vi "_Template Read sqlite configuration.vi"(8 "error in (no error)":errorcluster, 10 "Table in":string="employees", 11 "Configuration database in":path) -> (0 "error out":errorcluster, 1 "Values(str)":string[](array[string]), 2 "Names":string[](array[string]))   [LabVIEW 2020, in "sqlite3.lvlib" / "sqlite3.lvclass"]
uses:
  externals/sqlite3/Source/sqlite3.lvclass
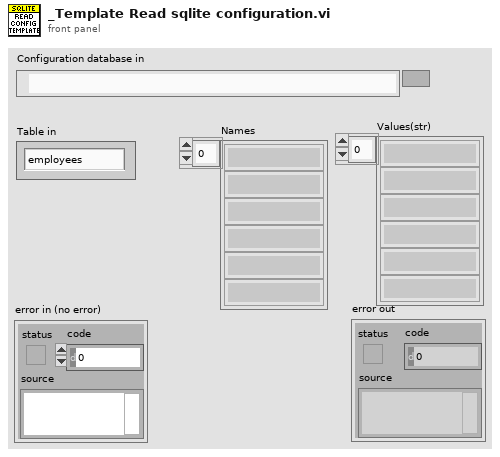
[diagram p1: front panel]
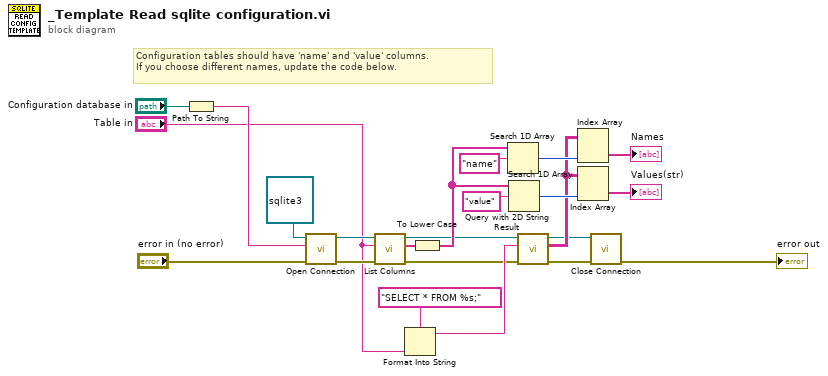
[diagram p0: block diagram]
diagram:
  # "Configuration tables should have 'name' and 'value' columns.\nIf you choose different names, update the code below."
  n1 = Path To String(path="Configuration database in") -> (string=w20:string)
  n2 = call-dynamic "Open Connection.vi"("error in (no error)"="error in (no error)", "DatabaseFilePath"=w20, "sqlite in"=refnum<class "sqlite3.lvclass"> refnum) -> ("error out"=w16:errorcluster, "sqlite out"=w17:refnum<class "sqlite3.lvclass">)  [unwired: 7 in]
  n3 = call-dynamic "List Columns.vi"("error in (no error)"=w16, "Table in"="Table in", "sqlite in"=w17) -> ("error out"=w4:errorcluster, "columns out"=w13:string[], "sqlite out"=w6:refnum<class "sqlite3.lvclass">)  [unwired: 5 in, 1 out]
  n4 = Format Into String(format string="SELECT * FROM %s;" ("sql (string)"), "Table in") -> (resulting string=w5:string)  [unwired: 2 in, 1 out]
  n5 = To Lower Case(string=w13) -> (all lower case string=w11:string[])
  n6 = Search 1D Array(1D array=w11, element="name" ("sql (string)")) -> (index of element=w10:i32)  [unwired: 1 in]
  n7 = Search 1D Array(1D array=w11, element="value" ("sql (string)")) -> (index of element=w9:i32)  [unwired: 1 in]
  n8 = call-dynamic "Query with 2D String Result.vi"("error in (no error)"=w4, "Query string"=w5, "sqlite3 in"=w6) -> ("error out"=w1:errorcluster, "Result"=w3:string[][], "sqlite3 out"=w2:refnum<class "sqlite3.lvclass">)  [unwired: 6 in]
  n9 = Index Array(array=w3, index (col)=w10) -> (element=→"Names":string[])  [unwired: 1 in]
  n10 = Index Array(array=w3, index (col)=w9) -> (element=→"Values(str)":string[])  [unwired: 1 in]
  n11 = call-dynamic "Close Connection.vi"("error in (no error)"=w1, "sqlite in"=w2) -> ("error out"=→"error out":errorcluster)  [unwired: 8 in, 1 out]
